vi "JSON text to Variant.vi"(8 "error in (no error)":errorcluster, 9 "Data Type":variant, 10 "Offset":i32, 11 "JSON":string) -> (0 "error out":errorcluster, 1 "Variant out":variant)   [LabVIEW 2017, in "JSONtext.lvlib"]
doc: "Convert JSON to the Data Type entered, which may be a cluster or array."
uses:
  JSONtext.lvlib
  <vilib>/Utility/Data Type/Type Definitions/Data Type.ctl
  JSON Value Type.ctl
  support/Get String.vi
  support/Get LVObject.vi
  support/Get Timestamp.vi
  support/Get I32.vi
  support/Get I64.vi
  support/Get U32.vi
  support/Get U64.vi
  support/Get Boolean.vi
  support/Get DBL.vi
  support/Get SGL.vi
  support/quote and escape json string 2.vi
  Parsing/Advance past String.vi
  support/Format Error.vi
  support/Get Number Text.vi
  Parsing/NaN or null to Integer ERROR.vi
  Parsing/Advance past Number.vi
  Parsing/Parsing Error.vi
  <vilib>/Utility/error.llb/Error Cluster From Error Code.vi
  <vilib>/Utility/Data Type/Get Numeric Information.vi
  support/Unescape JSON string.vi
  support/Scan Timestamp.vi
  <vilib>/Utility/Data Type/Get Refnum Information.vi
  <vilib>/Utility/Data Type/NI_Data Type.lvlib
  <vilib>/JDP Science/JDP Science Common Utilities/JDP Utility.lvlib
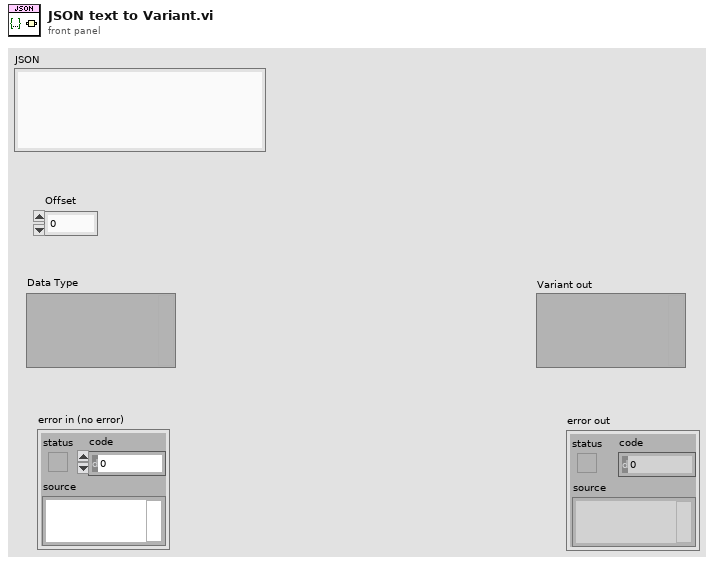
[diagram p1: front panel]
types:
  T1 = typedef "NI_Data Type.lvlib/Data Type.ctl" = enum8{"Invalid Type", "Void", "I8", "I16", "I32", "I64", "U8", "U16", "U32", "U64", "Single Float", "Double Float", "Extended Float", "Single Complex", "Double Complex", "Extended Complex", "Enum U8", "Enum U16", "Enum U32", "Enum U64", "Single Float With Unit", "Double Float With Unit", "Extended Float With Unit", "Single Complex with Unit", "Double Complex with Unit", "Extended Complex with Unit", "Boolean", "String", "Path", "Picture", "Tag", "Array", "Cluster", "Variant", "LV Variant", "Waveform", "Timestamp", "Digital Waveform", "Digital Data", "ExpressData", "Refnum", "External Data", "VI", "Poly VI", "LabVIEW Class Instance", "Fixed Point"}
  T2 = typedef "JSONtext.lvlib/Parsing State.ctl" = enum16{"Parser Error", "Object", "Array", "String", "Number/Other", "Leading Whitespace", "Object end", "Array end", "Value end"}
  T3 = typedef "JSONtext.lvlib/JSON Value Type.ctl" = enum16{"Not a JSON Value", "JSON Object", "JSON Array", "String", "Number", "true", "false", "null"}
  T4 = typedef "JSONtext.lvlib/Found Items.ctl" = cluster{"Item offset":i32, "Offset past Item":i32, "Name offset":i32, "Offset past Name":i32, "Found":bool, "Item Type":T2, "Item Index":i32}
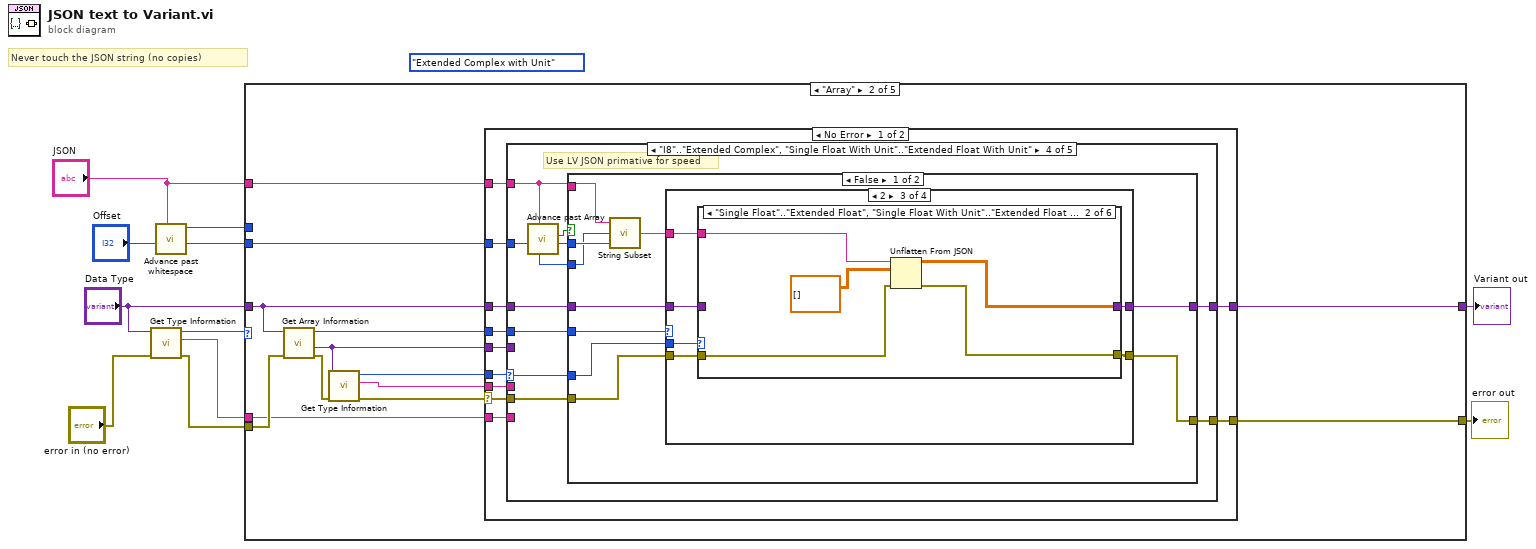
[diagram p0: block diagram]
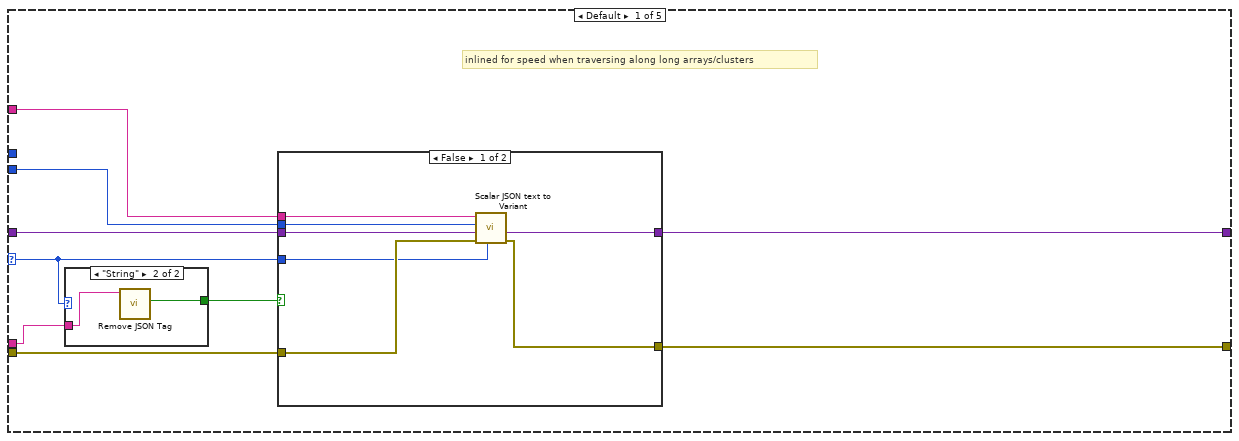
[diagram p2: hidden frame]
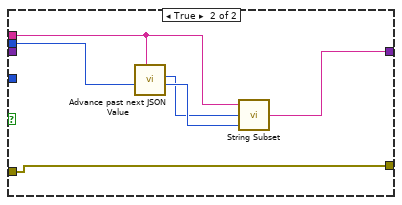
[diagram p3: hidden frame]
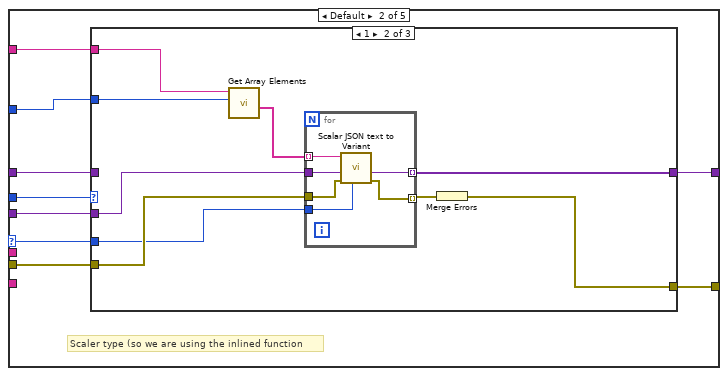
[diagram p6: hidden frame]
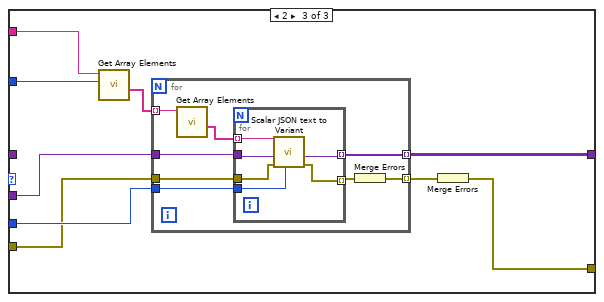
[diagram p8: hidden frame]
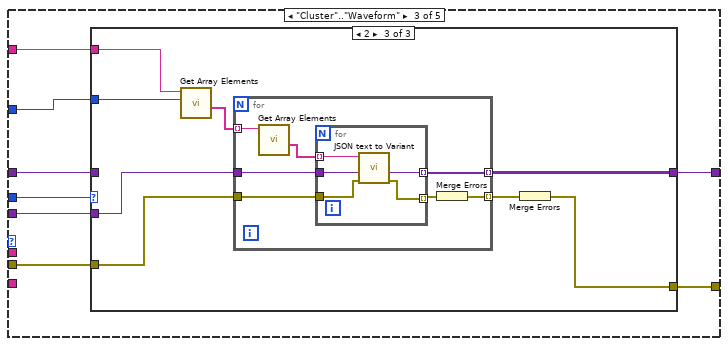
[diagram p9: hidden frame]
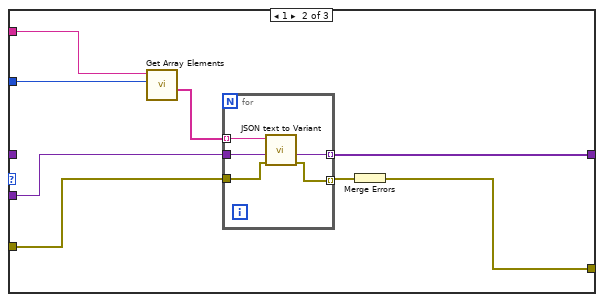
[diagram p11: hidden frame]
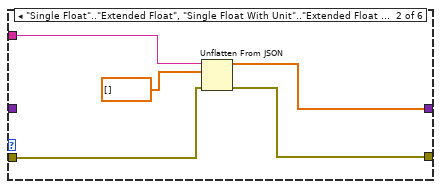
[diagram p14: hidden frame]
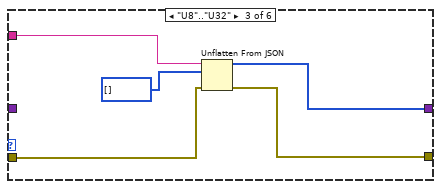
[diagram p15: hidden frame]
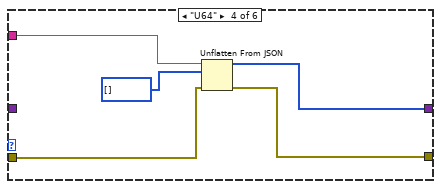
[diagram p16: hidden frame]
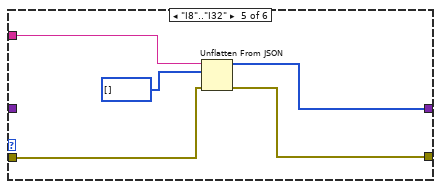
[diagram p17: hidden frame]
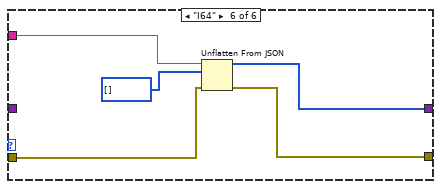
[diagram p18: hidden frame]
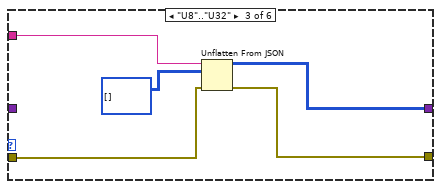
[diagram p20: hidden frame]
diagram:
  (unwired) Data_Type."Extended Complex with Unit" ("Type")
  # "Never touch the JSON string (no copies)"
  n1 = call <vilib>:"Get Type Information.vi"("error in (no error)"="error in (no error)", "Variant"="Data Type") -> ("error out"=w7:errorcluster, "Name"=w1:string, "Type"=w11:T1)  [unwired: 5 in, 2 out]
  n2 = call "Advance past whitespace.vi"("JSON"="JSON", "Offset"="Offset") -> ("Offset of first non-whitespace"=w4:i32, "Parser State"=w2:T2)  [unwired: 8 in]
  n3 = case shown="\"Array\"" w11 {
    selector: w11 -> [w13 _ _ _ _]
    tunnel: "Data Type" -> [w20 w41 w371 w384 w545]
    tunnel: "JSON" -> [w18 w39 w364 w376 w540]
    tunnel: [w15 w45 w361 w379 w537] -> w8
    tunnel: w7 -> [w16 w48 w370 w382 w544]
    tunnel: w4 -> [w17 w37 w363 w374 w539]
    tunnel: [w19 w44 w354 w380 w542] -> w6
    tunnel: w2 -> [_ _ _ _ _]
    tunnel: w1 -> [w14 w38 _ _ _]
    frame Default {
      # "inlined for speed when traversing along long arrays/clusters"
      n4 = case shown="\"String\"" w13 {
        tunnel: w14 -> [_ w35]
        tunnel: [_ w34] -> w12
        frame "Invalid Type", Default {
        }
        frame "String" {
          n5 = call "Remove JSON Tag.vi"("Name"=w35) -> ("tagged as JSON text"=w34:bool)  [unwired: 9 in, 1 out]
        }
      }
      n6 = case shown="False" w12 {
        tunnel: w20 -> [w27 _]
        tunnel: [w26 w29] -> w19
        tunnel: w18 -> [w25 w30]
        tunnel: w17 -> [w24 w33]
        tunnel: w16 -> [w23 w28]
        tunnel: [w22 w28] -> w15
        tunnel: w13 -> [w21 _]
        frame False {
          n7 = call "Scalar JSON text to Variant.vi"("Type"=w21, "error in (no error)"=w23, "Variant (Data Type)"=w27, "Offset"=w24, "JSON"=w25) -> ("error out"=w22:errorcluster, "Variant out"=w26:variant)  [unwired: 5 in]
        }
        frame True {
          n8 = call "Advance past next JSON Value.vi"("JSON"=w30, "Offset"=w33) -> ("Offset out"=w32:i32, "Value start"=w31:i32)  [unwired: 7 in, 1 out]
          n9 = call "String Subset.vi"("Offset past End"=w32, "Start offset"=w31, "JSON"=w30) -> ("substring"=w29:string)  [unwired: 2 in]
        }
      }
    }
    frame "Array" {
      n10 = call <vilib>:"Get Array Information.vi"("error in (no error)"=w48, "Variant"=w41) -> ("error out"=w47:errorcluster, "Array Element Data Type"=w40:variant, "Number of Dimensions"=w42:i32)  [unwired: 6 in, 1 out]
      n11 = call <vilib>:"Get Type Information.vi"("error in (no error)"=w47, "Variant"=w40) -> ("error out"=w46:errorcluster, "Name"=w36:string, "Type"=w43:T1)  [unwired: 5 in, 2 out]
      n12 = case shown="No Error" w46 {
        selector: w46 -> [w59 w353]
        tunnel: [w58 w353] -> w45
        tunnel: [w57 w352] -> w44
        tunnel: w43 -> [w56 _]
        tunnel: w42 -> [w55 _]
        tunnel: w41 -> [w54 w352]
        tunnel: w40 -> [w53 _]
        tunnel: w39 -> [w52 _]
        tunnel: w38 -> [w51 _]
        tunnel: w37 -> [w50 _]
        tunnel: w36 -> [w49 _]
        frame No Error {
          n13 = case shown="\"I8\"..\"Extended Complex\", \"Single Float With Unit\"..\"Extended Float With Unit\"" w56 {
            selector: w56 -> [_ w62 _ w159 _]
            tunnel: w52 -> [_ w66 w114 w157 w289]
            tunnel: w59 -> [w60 w69 w117 w164 w288]
            tunnel: [w60 w70 w118 w163 w287] -> w58
            tunnel: [w61 w67 w115 w162 w286] -> w57
            tunnel: w55 -> [_ w65 w113 w161 w285]
            tunnel: w54 -> [w61 w64 w112 w160 w284]
            tunnel: w53 -> [_ w68 w116 _ _]
            tunnel: w50 -> [_ w63 w111 w156 w281]
            tunnel: w51 -> [_ _ _ _ w283]
            tunnel: w49 -> [_ _ _ _ w280]
            frame "Invalid Type" {
            }
            frame Default {
              # "Scaler type (so we are using the inlined function"
              n14 = case shown="1" w65 {
                tunnel: [w71 w80 w90] -> w70
                tunnel: w69 -> [w71 w79 w88]
                tunnel: w68 -> [_ w78 w95]
                tunnel: [w72 w76 w93] -> w67
                tunnel: w63 -> [_ w75 w92]
                tunnel: w66 -> [_ w74 w91]
                tunnel: w64 -> [w72 _ _]
                tunnel: w62 -> [_ w73 w89]
                frame 0, Default {
                }
                frame 1 {
                  n15 = call "Get Array Elements.vi"("Offset"=w75, "JSON"=w74) -> ("<JSON>"=w77:string[])  [unwired: 7 in, 2 out]
                  n16 = for {
                    tunnel: w78 -> [w86]
                    tunnel: w79 -> [w84]
                    tunnel: [w83] -> w81 mode=indexing
                    tunnel: [w85] -> w76 mode=indexing
                    tunnel: w77 -> [w87] mode=indexing
                    tunnel: w73 -> [w82]
                    n17 = call "Scalar JSON text to Variant.vi"("Type"=w82, "error in (no error)"=w84, "Variant (Data Type)"=w86, "JSON"=w87) -> ("error out"=w83:errorcluster, "Variant out"=w85:variant)  [unwired: 6 in]
                  }
                  n18 = Merge Errors(w81) -> (w80:errorcluster)
                }
                frame 2 {
                  n19 = call "Get Array Elements.vi"("Offset"=w92, "JSON"=w91) -> ("<JSON>"=w94:string[])  [unwired: 7 in, 2 out]
                  n20 = for {
                    tunnel: [w103] -> w96 mode=indexing
                    tunnel: w88 -> [w102]
                    tunnel: w95 -> [w101]
                    tunnel: w94 -> [w99] mode=indexing
                    tunnel: [w100] -> w93 mode=indexing
                    tunnel: w89 -> [w97]
                    n21 = call "Get Array Elements.vi"("JSON"=w99) -> ("<JSON>"=w98:string[])  [unwired: 8 in, 2 out]
                    n22 = for {
                      tunnel: w101 -> [w106]
                      tunnel: w102 -> [w107]
                      tunnel: [w108] -> w104 mode=indexing
                      tunnel: [w109] -> w100 mode=indexing
                      tunnel: w98 -> [w110] mode=indexing
                      tunnel: w97 -> [w105]
                      n23 = call "Scalar JSON text to Variant.vi"("Type"=w105, "error in (no error)"=w107, "Variant (Data Type)"=w106, "JSON"=w110) -> ("error out"=w108:errorcluster, "Variant out"=w109:variant)  [unwired: 6 in]
                    }
                    n24 = Merge Errors(w104) -> (w103:errorcluster)
                  }
                  n25 = Merge Errors(w96) -> (w90:errorcluster)
                }
              }
            }
            frame "Cluster".."Waveform" {
              n26 = case shown="2" w113 {
                tunnel: [w119 w127 w134] -> w118
                tunnel: w117 -> [w119 w126 w140]
                tunnel: w116 -> [_ w125 w139]
                tunnel: [w120 w123 w137] -> w115
                tunnel: w111 -> [_ w122 w136]
                tunnel: w114 -> [_ w121 w135]
                tunnel: w112 -> [w120 _ _]
                frame 0, Default {
                }
                frame 1 {
                  n27 = call "Get Array Elements.vi"("Offset"=w122, "JSON"=w121) -> ("<JSON>"=w124:string[])  [unwired: 7 in, 2 out]
                  n28 = for {
                    tunnel: w125 -> [w133]
                    tunnel: w126 -> [w132]
                    tunnel: [w131] -> w128 mode=indexing
                    tunnel: [w130] -> w123 mode=indexing
                    tunnel: w124 -> [w129] mode=indexing
                    n29 = call "JSON text to Variant.vi"("error in (no error)"=w132, "Data Type"=w133, "JSON"=w129) -> ("error out"=w131:errorcluster, "Variant out"=w130:variant)  [unwired: 7 in]
                  }
                  n30 = Merge Errors(w128) -> (w127:errorcluster)
                }
                frame 2 {
                  n31 = call "Get Array Elements.vi"("Offset"=w136, "JSON"=w135) -> ("<JSON>"=w138:string[])  [unwired: 7 in, 2 out]
                  n32 = for {
                    tunnel: [w147] -> w141 mode=indexing
                    tunnel: w140 -> [w146]
                    tunnel: w139 -> [w145]
                    tunnel: w138 -> [w143] mode=indexing
                    tunnel: [w144] -> w137 mode=indexing
                    n33 = call "Get Array Elements.vi"("JSON"=w143) -> ("<JSON>"=w142:string[])  [unwired: 8 in, 2 out]
                    n34 = for {
                      tunnel: w145 -> [w153]
                      tunnel: w146 -> [w152]
                      tunnel: [w151] -> w148 mode=indexing
                      tunnel: [w150] -> w144 mode=indexing
                      tunnel: w142 -> [w149] mode=indexing
                      n35 = call "JSON text to Variant.vi"("error in (no error)"=w152, "Data Type"=w153, "JSON"=w149) -> ("error out"=w151:errorcluster, "Variant out"=w150:variant)  [unwired: 7 in]
                    }
                    n36 = Merge Errors(w148) -> (w147:errorcluster)
                  }
                  n37 = Merge Errors(w141) -> (w134:errorcluster)
                }
              }
            }
            frame "I8".."Extended Complex", "Single Float With Unit".."Extended Float With Unit" {
              # "Use LV JSON primative for speed"
              n38 = call "Advance past Array.vi"("JSON"=w157, "Offset"=w156) -> ("Offset past Array"=w158:i32, "Empty Array"=w154:bool, "Array Start"=w155:i32)  [unwired: 6 in, 1 out]
              n39 = case shown="False" w154 {
                tunnel: w164 -> [w174 w277]
                tunnel: [w173 w277] -> w163
                tunnel: [w172 w276] -> w162
                tunnel: w161 -> [w171 _]
                tunnel: w160 -> [w170 w276]
                tunnel: w159 -> [w168 _]
                tunnel: w158 -> [w167 _]
                tunnel: w157 -> [w166 _]
                tunnel: w155 -> [w165 _]
                frame False {
                  n40 = call "String Subset.vi"("Offset past End"=w167, "Start offset"=w165, "JSON"=w166) -> ("substring"=w169:string)  [unwired: 2 in]
                  n41 = case shown="2" w171 {
                    tunnel: w169 -> [_ w182 w215 w248]
                    tunnel: w174 -> [w175 w181 w214 w247]
                    tunnel: [w175 w180 w213 w246] -> w173
                    tunnel: [w176 w178 w211 w244] -> w172
                    tunnel: w170 -> [w176 w177 w210 w243]
                    tunnel: w168 -> [_ w179 w212 w245]
                    frame 0, Default {
                    }
                    frame 1 {
                      n42 = case shown="\"Invalid Type\", Default" w179 {
                        tunnel: w182 -> [_ w189 w194 w199 w204 w209]
                        tunnel: w181 -> [w183 w187 w192 w197 w202 w207]
                        tunnel: [w183 w186 w191 w196 w201 w206] -> w180
                        tunnel: [w184 w185 w190 w195 w200 w205] -> w178
                        tunnel: w177 -> [w184 _ _ _ _ _]
                        frame "Invalid Type", Default {
                        }
                        frame "Single Float".."Extended Float", "Single Float With Unit".."Extended Float With Unit" {
                          n43 = Unflatten From JSON(JSON string=w189, type and defaults=dbl[] [], error in (no error)=w187) -> (value=w185:dbl[], error out=w186:errorcluster)  [unwired: 4 in]
                        }
                        frame "U8".."U32" {
                          n44 = Unflatten From JSON(JSON string=w194, type and defaults=u32[] [], error in (no error)=w192) -> (value=w190:u32[], error out=w191:errorcluster)  [unwired: 4 in]
                        }
                        frame "U64" {
                          n45 = Unflatten From JSON(JSON string=w199, type and defaults=u64[] [], error in (no error)=w197) -> (value=w195:u64[], error out=w196:errorcluster)  [unwired: 4 in]
                        }
                        frame "I8".."I32" {
                          n46 = Unflatten From JSON(JSON string=w204, type and defaults=i32[] [], error in (no error)=w202) -> (value=w200:i32[], error out=w201:errorcluster)  [unwired: 4 in]
                        }
                        frame "I64" {
                          n47 = Unflatten From JSON(JSON string=w209, type and defaults=i64[] [], error in (no error)=w207) -> (value=w205:i64[], error out=w206:errorcluster)  [unwired: 4 in]
                        }
                      }
                    }
                    frame 2 {
                      n48 = case shown="\"Single Float\"..\"Extended Float\", \"Single Float With Unit\"..\"Extended Float With Unit\"" w212 {
                        tunnel: w215 -> [_ w222 w227 w232 w237 w242]
                        tunnel: w214 -> [w216 w220 w225 w230 w235 w240]
                        tunnel: [w216 w219 w224 w229 w234 w239] -> w213
                        tunnel: [w217 w218 w223 w228 w233 w238] -> w211
                        tunnel: w210 -> [w217 _ _ _ _ _]
                        frame "Invalid Type", Default {
                        }
                        frame "Single Float".."Extended Float", "Single Float With Unit".."Extended Float With Unit" {
                          n49 = Unflatten From JSON(JSON string=w222, type and defaults=dbl[][] [], error in (no error)=w220) -> (value=w218:dbl[][], error out=w219:errorcluster)  [unwired: 4 in]
                        }
                        frame "U8".."U32" {
                          n50 = Unflatten From JSON(JSON string=w227, type and defaults=u32[][] [], error in (no error)=w225) -> (value=w223:u32[][], error out=w224:errorcluster)  [unwired: 4 in]
                        }
                        frame "U64" {
                          n51 = Unflatten From JSON(JSON string=w232, type and defaults=u64[][] [], error in (no error)=w230) -> (value=w228:u64[][], error out=w229:errorcluster)  [unwired: 4 in]
                        }
                        frame "I8".."I32" {
                          n52 = Unflatten From JSON(JSON string=w237, type and defaults=i32[][] [], error in (no error)=w235) -> (value=w233:i32[][], error out=w234:errorcluster)  [unwired: 4 in]
                        }
                        frame "I64" {
                          n53 = Unflatten From JSON(JSON string=w242, type and defaults=i64[][] [], error in (no error)=w240) -> (value=w238:i64[][], error out=w239:errorcluster)  [unwired: 4 in]
                        }
                      }
                    }
                    frame 3 {
                      n54 = case shown="\"U8\"..\"U32\"" w245 {
                        tunnel: w248 -> [_ w255 w260 w265 w270 w275]
                        tunnel: w247 -> [w249 w253 w258 w263 w268 w273]
                        tunnel: [w249 w252 w257 w262 w267 w272] -> w246
                        tunnel: [w250 w251 w256 w261 w266 w271] -> w244
                        tunnel: w243 -> [w250 _ _ _ _ _]
                        frame "Invalid Type", Default {
                        }
                        frame "Single Float".."Extended Float", "Single Float With Unit".."Extended Float With Unit" {
                          n55 = Unflatten From JSON(JSON string=w255, type and defaults=dbl[][][] [], error in (no error)=w253) -> (value=w251:dbl[][][], error out=w252:errorcluster)  [unwired: 4 in]
                        }
                        frame "U8".."U32" {
                          n56 = Unflatten From JSON(JSON string=w260, type and defaults=u32[][][] [], error in (no error)=w258) -> (value=w256:u32[][][], error out=w257:errorcluster)  [unwired: 4 in]
                        }
                        frame "U64" {
                          n57 = Unflatten From JSON(JSON string=w265, type and defaults=u64[][][] [], error in (no error)=w263) -> (value=w261:u64[][][], error out=w262:errorcluster)  [unwired: 4 in]
                        }
                        frame "I8".."I32" {
                          n58 = Unflatten From JSON(JSON string=w270, type and defaults=i32[][][] [], error in (no error)=w268) -> (value=w266:i32[][][], error out=w267:errorcluster)  [unwired: 4 in]
                        }
                        frame "I64" {
                          n59 = Unflatten From JSON(JSON string=w275, type and defaults=i64[][][] [], error in (no error)=w273) -> (value=w271:i64[][][], error out=w272:errorcluster)  [unwired: 4 in]
                        }
                      }
                    }
                  }
                }
                frame True {
                }
              }
            }
            frame "String" {
              n60 = call "Remove JSON Tag.vi"("Name"=w280) -> ("tagged as JSON text"=w278:bool)  [unwired: 9 in, 1 out]
              n61 = call "Remove JSON Tag.vi"("Name"=w283) -> ("tagged as JSON text"=w282:bool)  [unwired: 9 in, 1 out]
              n62 = Or(x=w278, y=w282) -> (x .or. y?=w279:bool)
              n63 = case shown="True" w279 {
                tunnel: w289 -> [w296 w333]
                tunnel: w288 -> [w295 w332]
                tunnel: [w294 w331] -> w287
                tunnel: [w293 w330] -> w286
                tunnel: w285 -> [w292 w329]
                tunnel: w284 -> [w291 w328]
                tunnel: w281 -> [w290 w327]
                frame False {
                  # "#ds issue #2 Can't use LV primative\nbecause it mishandles zero bytes."
                  n64 = case shown="2" w292 {
                    tunnel: w296 -> [_ w303 w311]
                    tunnel: w295 -> [w297 w300 w312]
                    tunnel: [w297 w301 w313] -> w294
                    tunnel: [w298 w302 w314] -> w293
                    tunnel: w291 -> [w298 _ _]
                    tunnel: w290 -> [_ w299 w310]
                    frame 0, Default {
                    }
                    frame 1 {
                      n65 = call "Get Array Elements.vi"("error in (no error)"=w300, "Offset"=w299, "JSON"=w303) -> ("error out"=w305:errorcluster, "<JSON>"=w304:string[])  [unwired: 6 in, 1 out]
                      n66 = for {
                        tunnel: w304 -> [w309] mode=indexing
                        tunnel: [w308] -> w302 mode=indexing
                        shift-right: [w307] -> w301
                        shift-left: w305 -> [w306]
                        n67 = call "Strip Quotes and Unescape.vi"("error in (no error)"=w306, "String"=w309) -> ("error out"=w307:errorcluster, "result string"=w308:string)  [unwired: 8 in]
                      }
                    }
                    frame 2 {
                      n68 = call "Get Array Elements.vi"("error in (no error)"=w312, "Offset"=w310, "JSON"=w311) -> ("error out"=w316:errorcluster, "<JSON>"=w315:string[])  [unwired: 6 in, 1 out]
                      n69 = for {
                        tunnel: w315 -> [w322] mode=indexing
                        tunnel: [w319] -> w314 mode=indexing
                        shift-right: [w318] -> w313
                        shift-left: w316 -> [w321]
                        n70 = call "Get Array Elements.vi"("error in (no error)"=w321, "JSON"=w322) -> ("error out"=w317:errorcluster, "<JSON>"=w320:string[])  [unwired: 7 in, 1 out]
                        n71 = for {
                          tunnel: w320 -> [w326] mode=indexing
                          tunnel: [w325] -> w319 mode=indexing
                          shift-right: [w324] -> w318
                          shift-left: w317 -> [w323]
                          n72 = call "Strip Quotes and Unescape.vi"("error in (no error)"=w323, "String"=w326) -> ("error out"=w324:errorcluster, "result string"=w325:string)  [unwired: 8 in]
                        }
                      }
                    }
                  }
                }
                frame True {
                  # "JSON text"
                  n73 = case shown="1" w329 {
                    tunnel: w333 -> [_ w340 w342]
                    tunnel: w332 -> [w334 w339 w343]
                    tunnel: [w334 w338 w344] -> w331
                    tunnel: [w335 w337 w345] -> w330
                    tunnel: w328 -> [w335 _ _]
                    tunnel: w327 -> [_ w336 w341]
                    frame 0, Default {
                    }
                    frame 1 {
                      n74 = call "Get Array Elements.vi"("error in (no error)"=w339, "Offset"=w336, "JSON"=w340) -> ("error out"=w338:errorcluster, "<JSON>"=w337:string[])  [unwired: 6 in, 1 out]
                    }
                    frame 2 {
                      n75 = call "Get Array Elements.vi"("error in (no error)"=w343, "Offset"=w341, "JSON"=w342) -> ("error out"=w347:errorcluster, "<JSON>"=w346:string[])  [unwired: 6 in, 1 out]
                      n76 = for {
                        tunnel: w346 -> [w351] mode=indexing
                        tunnel: [w348] -> w345 mode=indexing
                        shift-right: [w349] -> w344
                        shift-left: w347 -> [w350]
                        n77 = call "Get Array Elements.vi"("error in (no error)"=w350, "JSON"=w351) -> ("error out"=w349:errorcluster, "<JSON>"=w348:string[])  [unwired: 7 in, 1 out]
                      }
                    }
                  }
                }
              }
            }
          }
        }
        frame Error {
        }
      }
    }
    frame "Waveform" {
      # "Attributes not supported"
      n78 = Variant To Data(error in=w370, type=waveform(dbl) {"t0"=timestamp(0 s since 1904-01-01), "dt"=1.0, "Y"=[]} ("waveform"), Variant=w371) -> (data=w368:waveform(dbl), error out=w362:errorcluster)
      n79 = Unbundle By Name(w368) -> ("t0"=w367:timestamp, "dt"=w366:dbl, "Y"=w365:dbl[])  [unwired: 1 out]
      n80 = Bundle("t0"=w367, "dt"=w366, "Y"=w365) -> (w359:cluster{"t0":timestamp, "dt":dbl, "Y":dbl[]})  [unwired: 1 in]
      n81 = call "JSON text to Variant.vi"("error in (no error)"=w362, "Data Type"=w359, "Offset"=w363, "JSON"=w364) -> ("error out"=w361:errorcluster, "Variant out"=w360:variant)  [unwired: 6 in]
      n82 = Variant To Data(type=w359, Variant=w360) -> (data=w358:cluster{"t0":timestamp, "dt":dbl, "Y":dbl[]})  [unwired: 1 in, 1 out]
      n83 = Unbundle By Name(w358) -> ("t0"=w357:timestamp, "dt"=w356:dbl, "Y"=w355:dbl[])
      n84 = Bundle By Name("t0"=w357, "dt"=w356, "Y"=w355) -> (w354:waveform(dbl))  [unwired: 1 in]
    }
    frame "Cluster" {
      n85 = Variant To Data(error in=w382, type=variant[] [], Variant=w384) -> (data=w372:variant[], error out=w378:errorcluster)
      n86 = Array Size(array=w372) -> (size(s)=w377:i32)
      n87 = case "Ragged Array?" shown="1" w377 {
        tunnel: w376 -> [_ w529]
        tunnel: [JSON_Value_Type."JSON Object" ("JSON Value Type") w528] -> w375
        tunnel: w374 -> [w519 w527]
        tunnel: [w519 w526] -> w373
        tunnel: w372 -> [_ w525]
        frame 0, Default {
        }
        frame 1 {
          n88 = Index Array(array=w525) -> (element=w524:variant)  [unwired: 1 in]
          n89 = call <vilib>:"Get Type Information.vi"("Variant"=w524) -> ("Type"=w523:T1)  [unwired: 6 in, 4 out]
          n90 = Equal?(x=Data_Type."Array", y=w523) -> (x = y?=w521:bool)
          n91 = case shown="True" w521 {
            tunnel: w529 -> [_ w535]
            tunnel: [JSON_Value_Type."JSON Object" ("JSON Value Type") w534] -> w528
            tunnel: w527 -> [w530 w533]
            tunnel: [w530 w532] -> w526
            frame False {
            }
            frame True {
              n92 = call "JSON type.vi"("Offset"=w533, "JSON"=w535) -> ("Item Offset"=w532:i32, "JSON Value Type"=w534:T3)  [unwired: 8 in]
            }
          }
        }
      }
      n93 = case shown="\"JSON Object\", Default" w375 {
        tunnel: [w395 w513] -> w381
        tunnel: [w394 w511] -> w379
        tunnel: w373 -> [w390 w515]
        tunnel: w378 -> [w389 w512]
        tunnel: w372 -> [w387 w518]
        tunnel: w376 -> [w386 w516]
        frame "JSON Object", Default {
          n94 = for {
            tunnel: w387 -> [w506] mode=indexing
            tunnel: w389 -> [w505]
            tunnel: [w504] -> w393 mode=indexing
            tunnel: [w502] -> w388 mode=indexing
            tunnel: [w503] -> w392 mode=indexing
            tunnel: [w500] -> w391 mode=indexing
            tunnel: [w496] -> w385
            i -> [w497]
            stop <- w496 stop-if-true
            n95 = call <vilib>:"Get Type Information.vi"("error in (no error)"=w505, "Variant"=w506) -> ("error out"=w504:errorcluster, "Name"=w501:string, "Type"=w502:T1)  [unwired: 5 in, 2 out]
            n96 = case shown="\"String\", \"Array\"" w502 {
              tunnel: w501 -> [w507 w510]
              tunnel: [_ w509] -> w503
              tunnel: [w507 w508] -> w499
              frame Default {
              }
              frame "String", "Array" {
                n97 = call "Remove JSON Tag.vi"("Name"=w510) -> ("tagged as JSON text"=w509:bool, "Name (tag stripped)"=w508:string)  [unwired: 9 in]
              }
            }
            n98 = Equal To 0?(x=w497) -> (x = 0?=w495:bool)
            n99 = Empty String/Path?(string/path=w499) -> (empty?=w498:bool)
            n100 = call "Quote and Escape JSON string.vi"("Plain Text"=w499) -> ("<JSON>"=w500:string)  [unwired: 10 in]
            n101 = And(x=w498, y=w495) -> (x .and. y?=w496:bool)
          }
          n102 = case shown="True" w385 {
            tunnel: [w408 w475] -> w395
            tunnel: [w407 w474] -> w394
            tunnel: w393 -> [w406 w478]
            tunnel: w392 -> [w404 _]
            tunnel: w391 -> [w403 _]
            tunnel: w390 -> [w402 w473]
            tunnel: w389 -> [w400 _]
            tunnel: w388 -> [w398 _]
            tunnel: w387 -> [w397 w477]
            tunnel: w386 -> [w396 w479]
            frame False {
              n103 = call "Find Object Item Locations by Names.vi"("Insertion point if not found"=TRUE, "Item Names <JSON>"=w403, "error in (no error)"=w400, "Object Offset"=w402, "JSON"=w396) -> ("error out"=w401:errorcluster, "Items"=w405:T4[])  [unwired: 5 in]
              n104 = for {
                tunnel: w397 -> [w420] mode=indexing
                tunnel: w396 -> [w419]
                tunnel: [w418] -> w409 mode=indexing
                tunnel: [w417] -> w408 mode=indexing
                tunnel: w406 -> [w416] mode=indexing
                tunnel: w398 -> [w415] mode=indexing
                tunnel: w405 -> [w414] mode=indexing
                tunnel: w404 -> [w410] mode=indexing
                n105 = Unbundle By Name(w414) -> ("Found"=w413:bool, "Item offset"=w412:i32, "Offset past Item"=w411:i32)
                n106 = case shown="True" w413 {
                  tunnel: w419 -> [_ w431]
                  tunnel: w412 -> [_ w430]
                  tunnel: w420 -> [w422 w429]
                  tunnel: [w422 w425] -> w417
                  tunnel: w416 -> [w421 w428]
                  tunnel: [w421 w427] -> w418
                  tunnel: w415 -> [_ w426]
                  tunnel: w411 -> [_ w423]
                  tunnel: w410 -> [_ w424]
                  frame False {
                  }
                  frame True {
                    n107 = case shown="True" w424 {
                      tunnel: w431 -> [w439 w460]
                      tunnel: w430 -> [w438 w459]
                      tunnel: w429 -> [w437 w453]
                      tunnel: w428 -> [w436 w455]
                      tunnel: [w435 w454] -> w427
                      tunnel: w426 -> [w432 w456]
                      tunnel: [w434 w457] -> w425
                      tunnel: w423 -> [_ w458]
                      frame False {
                        n108 = call "Is Scaler Type.vi"("Type"=w432) -> ("Scaler Type"=w433:bool)  [unwired: 2 in]
                        n109 = case shown="True" w433 {
                          tunnel: w439 -> [w446 w452]
                          tunnel: w438 -> [w445 w451]
                          tunnel: [w444 w450] -> w434
                          tunnel: w437 -> [w442 w449]
                          tunnel: w436 -> [w441 w448]
                          tunnel: [w443 w447] -> w435
                          tunnel: w432 -> [w440 _]
                          frame True {
                            n110 = call "Scalar JSON text to Variant.vi"("Type"=w440, "error in (no error)"=w441, "Variant (Data Type)"=w442, "Offset"=w445, "JSON"=w446) -> ("error out"=w443:errorcluster, "Variant out"=w444:variant)  [unwired: 5 in]
                          }
                          frame False {
                            n111 = call "JSON text to Variant.vi"("error in (no error)"=w448, "Data Type"=w449, "Offset"=w451, "JSON"=w452) -> ("error out"=w447:errorcluster, "Variant out"=w450:variant)  [unwired: 6 in]
                          }
                        }
                      }
                      frame True {
                        # "<JSON>"
                        n112 = case shown="\"Array\"" w456 {
                          tunnel: w460 -> [w466 w471]
                          tunnel: w459 -> [w465 w470]
                          tunnel: w458 -> [_ w469]
                          tunnel: [w462 w468] -> w457
                          tunnel: w455 -> [w463 w467]
                          tunnel: [w461 w467] -> w454
                          tunnel: w453 -> [w464 _]
                          frame "Array" {
                            n113 = call "JSON text to Variant.vi"("error in (no error)"=w463, "Data Type"=w464, "Offset"=w465, "JSON"=w466) -> ("error out"=w461:errorcluster, "Variant out"=w462:variant)  [unwired: 6 in]
                          }
                          frame "String", Default {
                            n114 = call "String Subset.vi"("Offset past End"=w469, "Start offset"=w470, "JSON"=w471) -> ("substring"=w468:string)  [unwired: 2 in]
                          }
                        }
                      }
                    }
                  }
                }
              }
              n115 = Merge Errors(w401, w409) -> (w407:errorcluster)
            }
            frame True {
              # "Unnamed cluster elements\n--> JSON Array"
              n116 = Merge Errors(w478) -> (w472:errorcluster)
              n117 = call "Get Array Elements.vi"("Offset"=w473, "JSON"=w479) -> ("<JSON>"=w476:string[])  [unwired: 7 in, 2 out]
              n118 = for {
                tunnel: w477 -> [w487] mode=indexing
                tunnel: w472 -> [w485]
                tunnel: [w484] -> w480 mode=indexing
                tunnel: [w486] -> w475 mode=indexing
                tunnel: w476 -> [w483]
                i -> [w481]
                n119 = Index Array(array=w483, index=w481) -> (element=w482:string)
                n120 = case shown="Default" w482 {
                  selector: w482 -> [_ w490]
                  tunnel: w487 -> [w489 w494]
                  tunnel: [w489 w493] -> w486
                  tunnel: w485 -> [w488 w492]
                  tunnel: [w488 w491] -> w484
                  frame "" {
                  }
                  frame Default {
                    n121 = call "JSON text to Variant.vi"("error in (no error)"=w492, "Data Type"=w494, "JSON"=w490) -> ("error out"=w491:errorcluster, "Variant out"=w493:variant)  [unwired: 7 in]
                  }
                }
              }
              n122 = Merge Errors(w480) -> (w474:errorcluster)
            }
          }
        }
        frame "JSON Array" {
          # "Let a JSON Array be valid for an Array as sole element in a Cluster, as this is a way of doing \"Ragged\" arrays in LabVIEW."
          n123 = Index Array(array=w518) -> (element=w517:variant)  [unwired: 1 in]
          n124 = call "JSON text to Variant.vi"("error in (no error)"=w512, "Data Type"=w517, "Offset"=w515, "JSON"=w516) -> ("error out"=w511:errorcluster, "Variant out"=w514:variant)  [unwired: 6 in]
          n125 = Build Array(w514) -> (w513:variant[])
        }
      }
      n126 = call <vilib>:"Array of Variants to Cluster.vi"("Array of Variants"=w381) -> ("Cluster of Variants"=w380:variant)  [unwired: 10 in]
    }
    frame "Variant", "LV Variant" {
      # "Unwrap and rewrap"
      n127 = Variant To Data(error in=w544, type=variant, Variant=w545) -> (data=w536:variant, error out=w541:errorcluster)
      n128 = call "JSON text to Variant.vi"("error in (no error)"=w541, "Data Type"=w536, "Offset"=w539, "JSON"=w540) -> ("error out"=w537:errorcluster, "Variant out"=w538:variant)  [unwired: 6 in]
      n129 = To Variant(anything=w538) -> (Variant=w542:variant)
    }
  }
  "Variant out" <- w6
  "error out" <- w8
